vi "T'触发器(调用自动翻转).vi"(2 "error in (no error)":errorcluster caption="错误输入（无错误）") -> (0 "error out":errorcluster caption="错误输出", 1 "Q":bool)   [LabVIEW 2012]
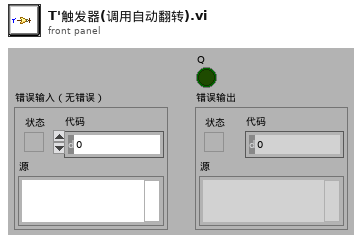
[diagram p1: front panel]
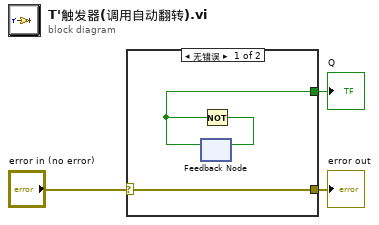
[diagram p0: block diagram]
diagram:
  n1 = case shown="无错误" "error in (no error)" {
    selector: "error in (no error)" -> [w6 w7]
    tunnel: [w6 w7] -> w2
    tunnel: [w4 _] -> w1
    frame No Error {
      n2 = feedback #1() -> (w4:bool)  [unwired: 1 in]
      n3 = Not(x=w4) -> (.not. x?=w5:bool)
      n4 = feedback-in #1(w5) -> ()
    }
    frame Error {
    }
  }
  "error out" <- w2
  "Q" <- w1
